vi "Parse Message From Websockets.vi"(8 "Error In":errorcluster) -> (0 "error out":errorcluster)   [LabVIEW 2014]
uses:
  Globals/messages.vi
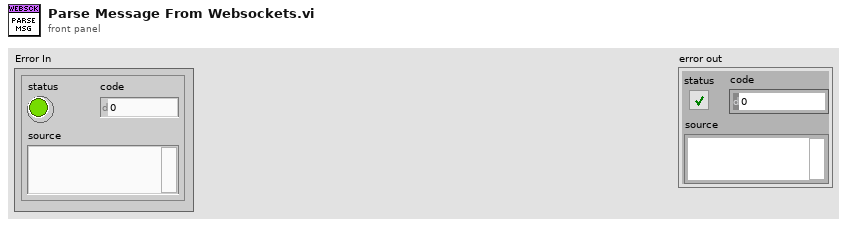
[diagram p1: front panel]
types:
  T1 = typedef "Websocket Data.ctl" = cluster{"Command":string, "Data":string}
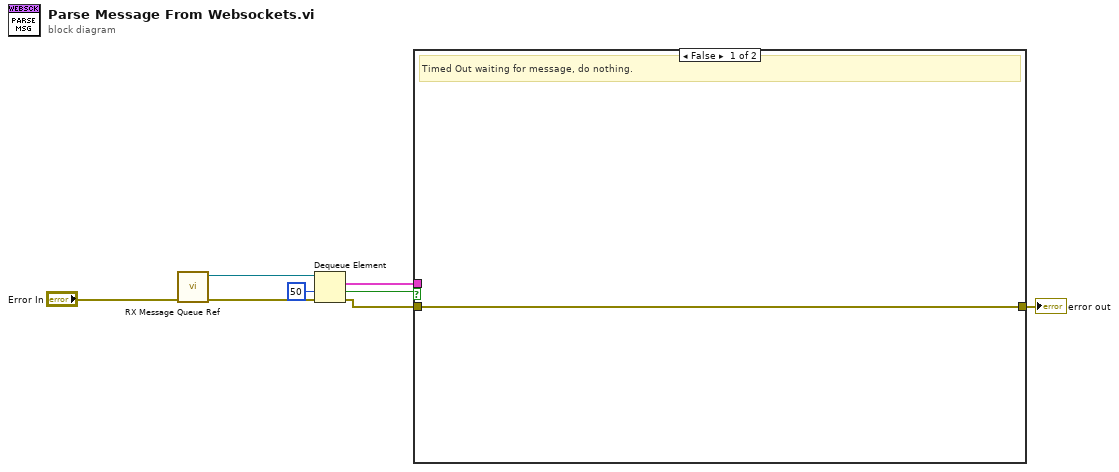
[diagram p0: block diagram]
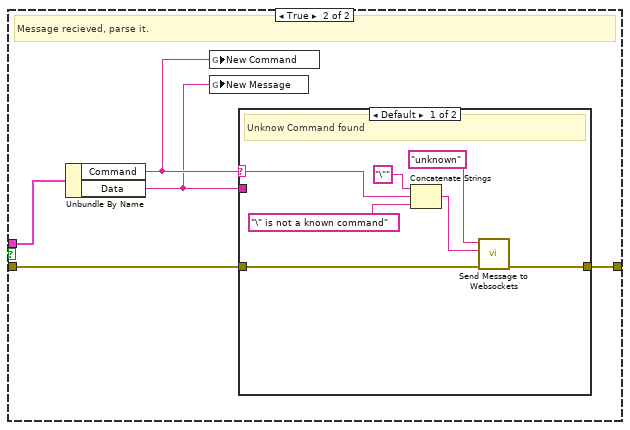
[diagram p2: hidden frame]
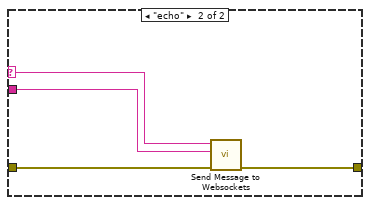
[diagram p3: hidden frame]
diagram:
  n1 = call "RX Message Queue Ref.vi"("Error In"="Error In") -> ("error out"=w8:errorcluster, "rx queue ref"=w7:refnum<queue>)  [unwired: 9 in]
  n2 = Dequeue Element(queue=w7, timeout in ms (-1)=50, error in (no error)=w8) -> (element=w3:T1, timed out?=w4:bool, error out=w2:errorcluster)  [unwired: 1 out]
  n3 = case shown="False" w4 {
    tunnel: w3 -> [_ w14]
    tunnel: w2 -> [w9 w11]
    tunnel: [w9 w10] -> w1
    frame False {
      # "Timed Out waiting for message, do nothing."
    }
    frame True {
      # "Message recieved, parse it."
      n4 = Unbundle By Name(w14) -> ("Command"=w13:string, "Data"=w12:string)
      n5 = global write "messages.vi" "New Command"(w13) -> ()
      n6 = global write "messages.vi" "New Message"(w12) -> ()
      n7 = case shown="Default" w13 {
        selector: w13 -> [w18 w24]
        tunnel: w12 -> [_ w23]
        tunnel: w11 -> [w20 w25]
        tunnel: [w21 w22] -> w10
        frame Default {
          # "Unknow Command found"
          n8 = Concatenate Strings("\"" ("string"), w18, "\" is not a known command" ("string")) -> (w15:string)
          n9 = call "Send Message to Websockets.vi"("Error In"=w20, "Data"=w15, "Command"="unknown") -> ("error out"=w21:errorcluster)  [unwired: 8 in]
        }
        frame "echo" {
          n10 = call "Send Message to Websockets.vi"("Error In"=w25, "Data"=w23, "Command"=w24) -> ("error out"=w22:errorcluster)  [unwired: 8 in]
        }
      }
    }
  }
  "error out" <- w1
